vi "midterm.vi"() -> ()   [LabVIEW 2022 SP3]
uses:
  <vilib>/express/express analysis/Spectral/Block/exnSpectralBlock spectral measurements RMS poly.vi
  <vilib>/express/express analysis/Spectral/Block/exnSpectralBlock spectral measurements RMS DDT.vi
  <vilib>/express/express analysis/Spectral/XNode/ExpressSpectralMeasurementsBlockNode.xnode
panel:
  in  "?":bool
  out "Input Signal":dynamicdata(graph) caption="Data"
  out "Input Spectrum":dynamicdata(graph)
  in  "Duration of\nCollection (s)":dbl=1.0 caption="Duration (s)"
  out "Frequency of Note":dbl[](array[numeric]) format="%.2p"
  out "Note Detected":string
  in  "?":bool
  in  "stop":bool
  # "Find Fundamental Frequency"
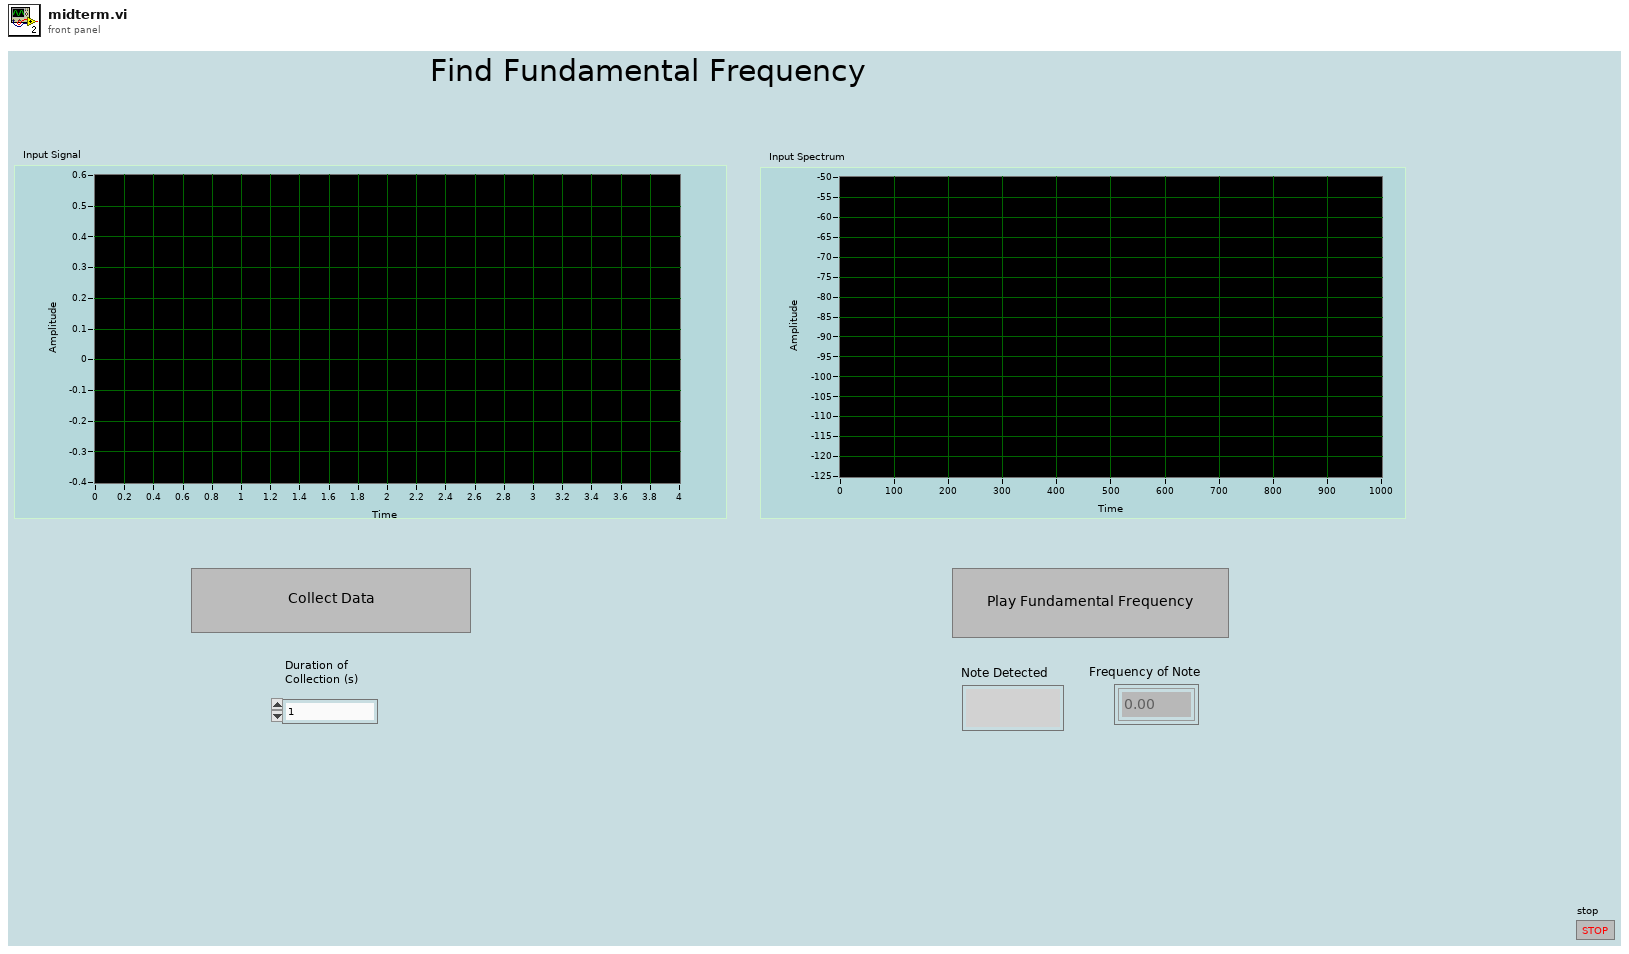
[diagram p1: front panel]
types:
  T1 = cluster{"averaging mode":u16, "weighting mode":u16, "number of averages":u32}
  T2 = cluster{"dB On (F)":bool, "unwrap phase (F)":bool, "convert to degree (F)":bool}
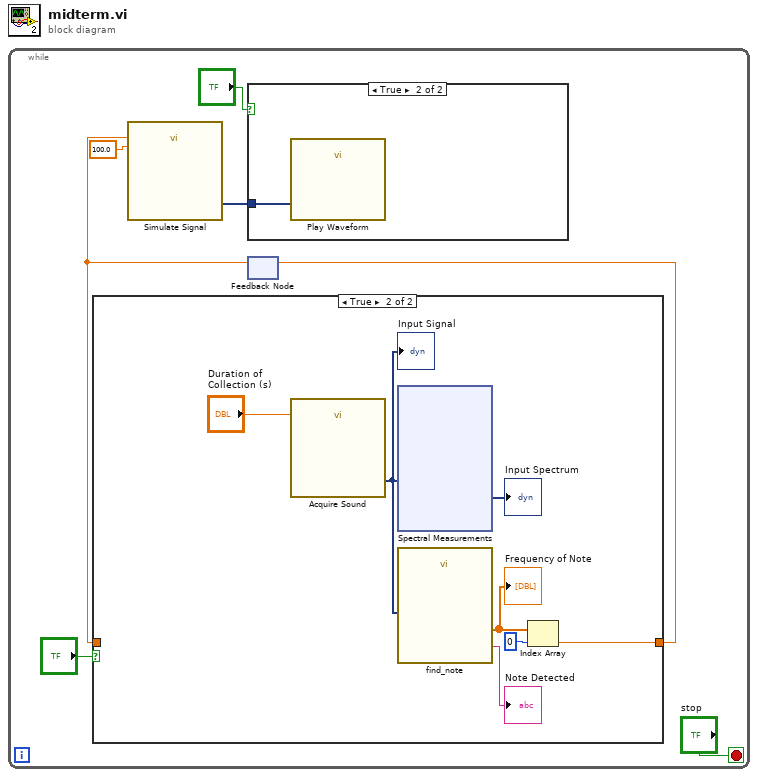
[diagram p0: block diagram]
diagram:
  n1 = while {
    stop <- "stop" stop-if-true
    n2 = feedback #1() -> (w1:dbl)  [unwired: 1 in]
    n3 = case shown="True" "?" {
      tunnel: [w9 w10] -> w2
      tunnel: w1 -> [w9 _]
      frame False {
      }
      frame True {
        n4 = call "Acquire Sound"("Duration (s)"="Duration of\nCollection (s)") -> ("Data"=w14:dynamicdata)  [unwired: 17 in, 1 out]
        "Input Signal" <- w14
        n5 = xnode "Spectral Measurements"("Signals"=w14) -> ("FFT - (RMS)"=→"Input Spectrum":dynamicdata)  [unwired: 1 in, 2 out]
        n6 = call "find_note.vi"("Data"=w14) -> ("Note"=→"Note Detected":string, "Frequency"=w11:dbl[])  [unwired: 9 in]
        "Frequency of Note" <- w11
        n7 = Index Array(array=w11, index=0) -> (element=w10:dbl)
      }
    }
    n8 = call "Simulate Signal"("Frequency"=w1, "Amplitude"=100.0) -> ("Sine"=w4:dynamicdata)  [unwired: 12 in, 1 out]
    n9 = case shown="True" "?" {
      tunnel: w4 -> [_ w8]
      frame False {
      }
      frame True {
        n10 = call "Play Waveform"("Data"=w8) -> ()  [unwired: 18 in, 1 out]
      }
    }
    n11 = feedback-in #1(w2) -> ()
  }
